vi "Begin.vi"(8 "error in":errorcluster) -> (0 "error out":errorcluster)   [LabVIEW 2018]
doc: "Called before other user functions, this VI is expected to open initial I/O refnums, load in file data, and do all program initialization. Notice that the <B>error out</B> terminal is simply used for data flow. Wiring it to other structures or subVIs ensures that this VI runs first."
uses:
  <vilib>/Rock Robotics/WPI/DriverStation/WPI_DriverStationRobotMode2.ctl
  <vilib>/Rock Robotics/WPI/Joystick/WPI_JoystickDeviceEnum.ctl
  <vilib>/Rock Robotics/WPI/Solenoid/WPI_SolenoidChannel.ctl
  <vilib>/Rock Robotics/WPI/ThirdParty/Phoenix-LabVIEW/Motor Controller/Controls/CTRE_Phoenix_MotorControl_NeutralMode.ctl
  <vilib>/Rock Robotics/WPI/ThirdParty/REV Robotics/SPARK MAX/Typedef/Spark MAX Idle Mode.ctl
  Robot Global Data.vi
  <vilib>/Rock Robotics/Network Tables/NT Write String Array.vi
  <vilib>/Rock Robotics/WPI/Solenoid/WPI_SolenoidOpenDouble.vi
  <vilib>/Rock Robotics/WPI/Solenoid/WPI_SolenoidOpenSingle.vi
  <vilib>/Rock Robotics/WPI/Utilities/WPI_GetSetVariantRefNum.vi
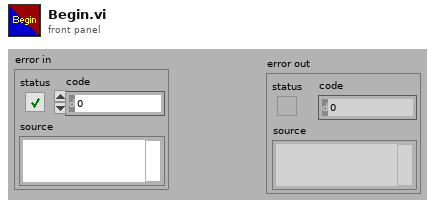
[diagram p1: front panel]
types:
  T1 = typedef "WPI_SolenoidChannel.ctl" = enum8{"Solenoid 0", "Solenoid 1", "Solenoid 2", "Solenoid 3", "Solenoid 4", "Solenoid 5", "Solenoid 6", "Solenoid 7", "Invalid"}
  T2 = typedef "Spark MAX Idle Mode.ctl" = enum16{"Coast", "Brake"}
  T3 = typedef "CTRE_Phoenix_MotorControl_NeutralMode.ctl" = enum8{"EEPROMSetting", "Override to Coast", "Override to Brake"}
  T4 = typedef "WPI_JoystickDeviceEnum.ctl" = enum16{"USB 0", "USB 1", "USB 2", "USB 3", "USB 4", "USB 5"}
  T5 = typedef "WPI_DriverStationRobotMode2.ctl" = enum16{"Autonomous Disabled", "Autonomous Enabled", "Teleop Disabled", "Teleop Enabled", "Disconnected", "Finish", "Test Disabled", "Test Enabled", "Emergency Stopped"}
  T6 = typedef "WPI_JoystickDevRef.ctl" = cluster{"Device":T4}
  T7 = typedef "WPI_MotorControlDeviceRef.ctl" = cluster{"DeviceStatus":errorcluster, "Type":T8, "PWM":cluster{"PWM Channel":T9, "DeadBand":T10}, "CAN":cluster{"Device Number":u8, "SetOutput VI Ref":variant, "GetOutput VI Ref":variant, "Enable VI Ref":variant, "Disable VI Ref":variant, "Data":variant}, "Invert":bool, "DIO PWM":cluster{"PWM \"Enable\" Channel":T9, "DIOChannel":T11, "PWM Rate":dbl}}
  T8 = typedef "WPI_MotorControlType.ctl" = enum16{"PWM", "CAN", "DIO PWM"}
  T9 = typedef "FPGA_DIOPWMChannel.ctl" = enum8{"PWM 0", "PWM 1", "PWM 2", "PWM 3", "PWM 4", "PWM 5", "PWM 6", "PWM 7", "PWM 8", "PWM 9", "PWM MXP 0", "PWM MXP 1", "PWM MXP 2", "PWM MXP 3", "PWM MXP 4", "PWM MXP 5", "PWM MXP 6", "PWM MXP 7", "PWM MXP 8", "PWM MXP 9", "Invalid"}
  T10 = typedef "WPI_PWMDeadband.ctl" = cluster{"Name":string, "maxPositivePwm":i32, "minPositivePwm":i32, "centerPwm":i32, "maxNegativePwm":i32, "minNegativePwm":i32, "angularRange":u16}
  T11 = typedef "FPGA_DIOChannel.ctl" = enum8{"DIO 0", "DIO 1", "DIO 2", "DIO 3", "DIO 4", "DIO 5", "DIO 6", "DIO 7", "DIO 8", "DIO 9", "DIO MXP 0", "DIO MXP 1", "DIO MXP 2", "DIO MXP 3", "DIO MXP 4", "DIO MXP 5", "DIO MXP 6", "DIO MXP 7", "DIO MXP 8", "DIO MXP 9", "DIO MXP 10", "DIO MXP 11", "DIO MXP 12", "DIO MXP 13", "DIO MXP 14", "DIO MXP 15", "SPI Port CS1", "SPI Port CS2", "SPI Port CS3", "SPI Port MISO", "SPI Port MOSI", "Invalid"}
  T12 = typedef "WPI_CompressorDevRef.ctl" = cluster{"DevStatus":errorcluster, "Pneumatics Control Module":u8}
  T13 = typedef "WPI_SolenoidDevRef.ctl" = cluster{"DevStatus":errorcluster, "Pneumatics Control Module":u8, "Forward Solenoid Channel":T1, "Reverse Solenoid Channel":T1}
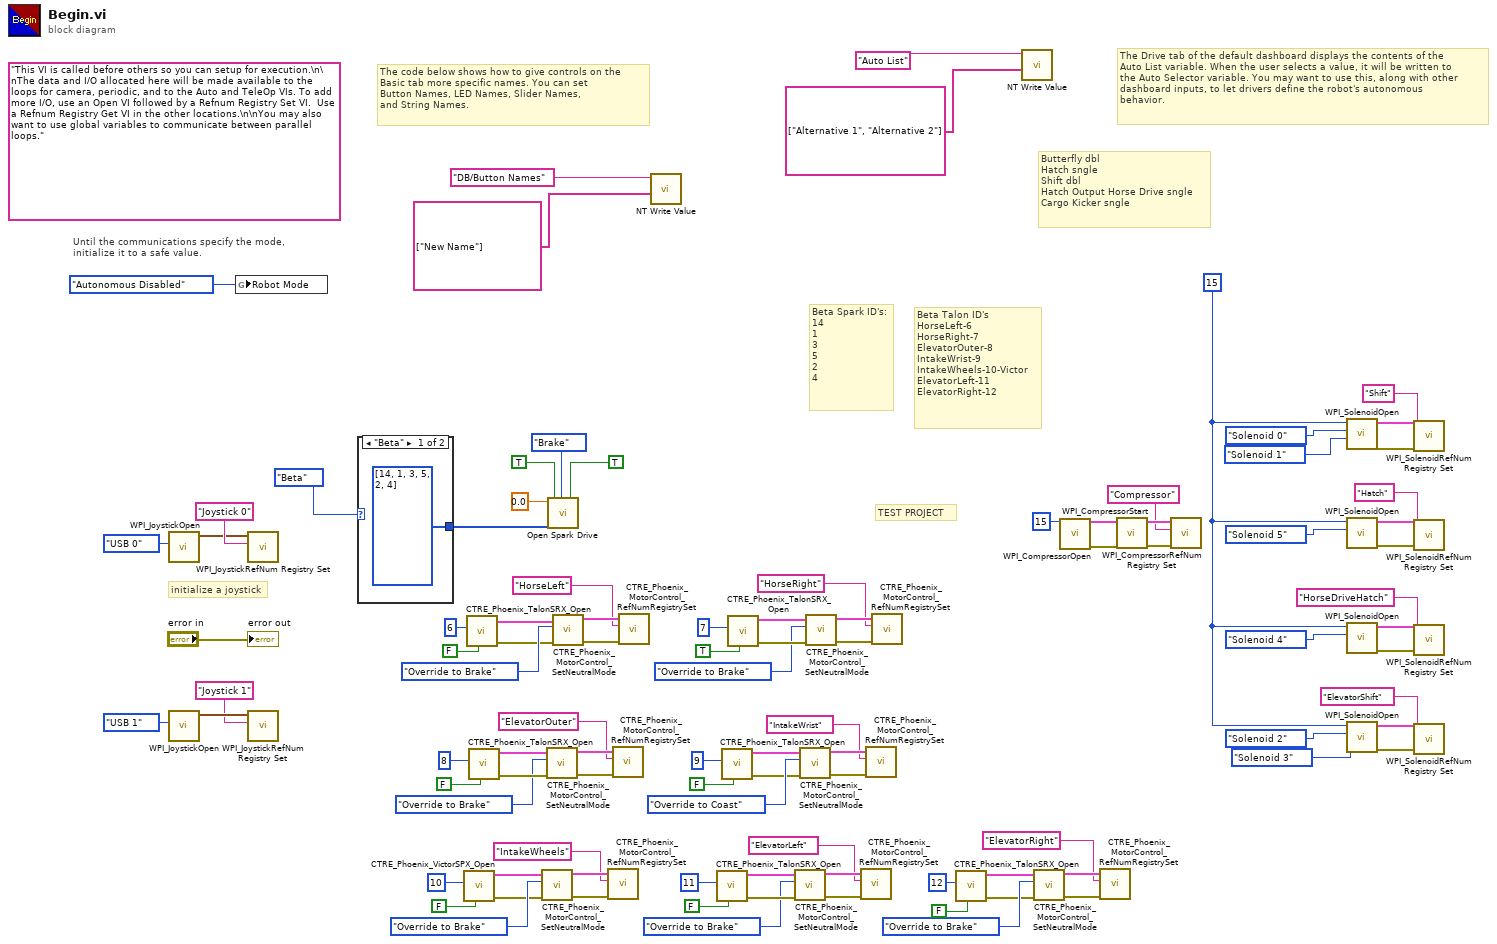
[diagram p0: block diagram]
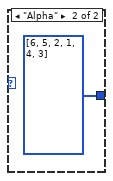
[diagram p2: hidden frame]
diagram:
  w77 = u8 15 ("Pneumatics Control Module (0)")
  (unwired) "This VI is called before others so you can setup for execution.\n\nThe data and I/O allocated here will be made available to the loops for camera, periodic, and to the Auto and TeleOp VIs. To add more I/O, use an Open VI followed by a Refnum Registry Set VI.  Use a Refnum Registry Get VI in the other locations.\n\nYou may also want to use global variables to communicate between parallel loops."
  # "Beta Talon ID's\nHorseLeft-6\nHorseRight-7\nElevatorOuter-8\nIntakeWrist-9\nIntakeWheels-10-Victor\nElevatorLeft-11\nElevatorRight-12"
  # "Beta Spark ID's:\n14\n1\n3\n5\n2\n4"
  # "TEST PROJECT"
  # "Butterfly dbl \nHatch sngle\nShift dbl\nHatch Output Horse Drive sngle\nCargo Kicker sngle"
  # "The Drive tab of the default dashboard displays the contents of the\nAuto List variable. When the user selects a value, it will be written to\nthe Auto Selector variable. You may want to use this, along with other\ndashboard inputs, to let drivers define the robot's autonomous\nbehavior."
  # "The code below shows how to give controls on the\nBasic tab more specific names. You can set\nButton Names, LED Names, Slider Names,\nand String Names."
  # "initialize a joystick"
  # "Until the communications specify the mode,\ninitialize it to a safe value."
  n1 = call <vilib>:"WPI_JoystickOpen.vi"("JoystickDevice"=WPI_JoystickDeviceEnum."USB 0") -> ("JoystickDevRef"=w97:T6)  [unwired: 10 in]
  n2 = call <vilib>:"WPI_JoystickOpen.vi"("JoystickDevice"=WPI_JoystickDeviceEnum."USB 1") -> ("JoystickDevRef"=w75:T6)  [unwired: 10 in]
  n3 = global write "Robot Global Data.vi" "Robot Mode"(WPI_DriverStationRobotMode2."Autonomous Disabled" ("Robot Mode")) -> ()
  n4 = call <vilib>:"WPI_JoystickRefNum Registry Set.vi"("refnum name"="Joystick 0", "JoystickDevRef"=w97) -> ()  [unwired: 8 in, 2 out]
  n5 = call <vilib>:"WPI_JoystickRefNum Registry Set.vi"("refnum name"="Joystick 1", "JoystickDevRef"=w75) -> ()  [unwired: 8 in, 2 out]
  n6 = case shown="\"Beta\"" enum16{"Alpha", "Beta"}."Beta" {
    tunnel: [u8[] [14, 1, 3, 5, 2, 4] ("CAN IDs") u8[] [6, 5, 2, 1, 4, 3] ("CAN IDs")] -> w2
    frame "Beta" {
    }
    frame "Alpha" {
    }
  }
  n7 = call <vilib>:"CTRE_Phoenix_VictorSPX_Open.vi"("Invert"=FALSE, "Device Number"=u8 10) -> ("error out"=w52:errorcluster, "CAN Talon SRX Ref"=w53:T7)  [unwired: 8 in]
  n8 = call <vilib>:"CTRE_Phoenix_TalonSRX_Open.vi"("Invert"=FALSE, "Device Number"=u8 6) -> ("error out"=w18:errorcluster, "CAN Talon SRX Ref"=w19:T7)  [unwired: 8 in]
  n9 = call <vilib>:"CTRE_Phoenix_TalonSRX_Open.vi"("Invert"=FALSE, "Device Number"=u8 8) -> ("error out"=w57:errorcluster, "CAN Talon SRX Ref"=w56:T7)  [unwired: 8 in]
  n10 = call <vilib>:"CTRE_Phoenix_MotorControl_SetNeutralMode.vi"("error in (no error)"=w52, "Motor Control Neutral Mode"=CTRE_Phoenix_MotorControl_NeutralMode."Override to Brake", "PhoenixMotorControlDevRef"=w53) -> ("error out"=w50:errorcluster, "PhoenixMotorControlDevRef"=w51:T7)  [unwired: 7 in]
  n11 = call <vilib>:"CTRE_Phoenix_MotorControl_SetNeutralMode.vi"("error in (no error)"=w57, "Motor Control Neutral Mode"=CTRE_Phoenix_MotorControl_NeutralMode."Override to Brake", "PhoenixMotorControlDevRef"=w56) -> ("error out"=w59:errorcluster, "PhoenixMotorControlDevRef"=w58:T7)  [unwired: 7 in]
  n12 = call "Open Spark Drive.vi"("Set Master/Slave?"=TRUE, "Set Ramp Rate?"=TRUE, "CAN IDs"=w2, "Idle Mode"=Spark_MAX_Idle_Mode."Brake", "Full Acceleration Time"=sgl 0.0 ("Seconds from neutral to full (0)")) -> ()  [unwired: 7 in]
  n13 = call <vilib>:"CTRE_Phoenix_MotorControl_SetNeutralMode.vi"("error in (no error)"=w18, "Motor Control Neutral Mode"=CTRE_Phoenix_MotorControl_NeutralMode."Override to Brake", "PhoenixMotorControlDevRef"=w19) -> ("error out"=w62:errorcluster, "PhoenixMotorControlDevRef"=w63:T7)  [unwired: 7 in]
  n14 = call <vilib>:"CTRE_Phoenix_MotorControl_RefNumRegistrySet.vi"("error in (no error)"=w50, "refnum name"="IntakeWheels" ("string"), "PhoenixMotorControlDevRef"=w51) -> ()  [unwired: 7 in, 2 out]
  n15 = call <vilib>:"CTRE_Phoenix_MotorControl_RefNumRegistrySet.vi"("error in (no error)"=w59, "refnum name"="ElevatorOuter" ("string"), "PhoenixMotorControlDevRef"=w58) -> ()  [unwired: 7 in, 2 out]
  n16 = call <vilib>:"CTRE_Phoenix_MotorControl_RefNumRegistrySet.vi"("error in (no error)"=w62, "refnum name"="HorseLeft" ("string"), "PhoenixMotorControlDevRef"=w63) -> ()  [unwired: 7 in, 2 out]
  n17 = call-poly <vilib>:"NT Write Value.vi"("String Array"=string[] ["New Name"], "Name"="DB/Button Names") -> ()  [unwired: 9 in, 1 out]
  n18 = call <vilib>:"CTRE_Phoenix_TalonSRX_Open.vi"("Invert"=FALSE, "Device Number"=u8 11) -> ("error out"=w43:errorcluster, "CAN Talon SRX Ref"=w42:T7)  [unwired: 8 in]
  n19 = call <vilib>:"CTRE_Phoenix_TalonSRX_Open.vi"("Invert"=FALSE, "Device Number"=u8 9) -> ("error out"=w38:errorcluster, "CAN Talon SRX Ref"=w39:T7)  [unwired: 8 in]
  n20 = call <vilib>:"CTRE_Phoenix_TalonSRX_Open.vi"("Invert"=TRUE, "Device Number"=u8 7) -> ("error out"=w29:errorcluster, "CAN Talon SRX Ref"=w28:T7)  [unwired: 8 in]
  n21 = call <vilib>:"CTRE_Phoenix_MotorControl_SetNeutralMode.vi"("error in (no error)"=w43, "Motor Control Neutral Mode"=CTRE_Phoenix_MotorControl_NeutralMode."Override to Brake", "PhoenixMotorControlDevRef"=w42) -> ("error out"=w45:errorcluster, "PhoenixMotorControlDevRef"=w44:T7)  [unwired: 7 in]
  n22 = call <vilib>:"CTRE_Phoenix_MotorControl_SetNeutralMode.vi"("error in (no error)"=w38, "Motor Control Neutral Mode"=CTRE_Phoenix_MotorControl_NeutralMode."Override to Coast", "PhoenixMotorControlDevRef"=w39) -> ("error out"=w36:errorcluster, "PhoenixMotorControlDevRef"=w37:T7)  [unwired: 7 in]
  n23 = call <vilib>:"CTRE_Phoenix_MotorControl_SetNeutralMode.vi"("error in (no error)"=w29, "Motor Control Neutral Mode"=CTRE_Phoenix_MotorControl_NeutralMode."Override to Brake", "PhoenixMotorControlDevRef"=w28) -> ("error out"=w31:errorcluster, "PhoenixMotorControlDevRef"=w30:T7)  [unwired: 7 in]
  n24 = call <vilib>:"CTRE_Phoenix_MotorControl_RefNumRegistrySet.vi"("error in (no error)"=w45, "refnum name"="ElevatorLeft" ("string"), "PhoenixMotorControlDevRef"=w44) -> ()  [unwired: 7 in, 2 out]
  n25 = call <vilib>:"CTRE_Phoenix_MotorControl_RefNumRegistrySet.vi"("error in (no error)"=w36, "refnum name"="IntakeWrist" ("string"), "PhoenixMotorControlDevRef"=w37) -> ()  [unwired: 7 in, 2 out]
  n26 = call <vilib>:"CTRE_Phoenix_MotorControl_RefNumRegistrySet.vi"("error in (no error)"=w31, "refnum name"="HorseRight" ("string"), "PhoenixMotorControlDevRef"=w30) -> ()  [unwired: 7 in, 2 out]
  n27 = call <vilib>:"CTRE_Phoenix_TalonSRX_Open.vi"("Invert"=FALSE, "Device Number"=u8 12) -> ("error out"=w24:errorcluster, "CAN Talon SRX Ref"=w25:T7)  [unwired: 8 in]
  n28 = call-poly <vilib>:"NT Write Value.vi"("String Array"=string[] ["Alternative 1", "Alternative 2"], "Name"="Auto List") -> ()  [unwired: 9 in, 1 out]
  n29 = call <vilib>:"CTRE_Phoenix_MotorControl_SetNeutralMode.vi"("error in (no error)"=w24, "Motor Control Neutral Mode"=CTRE_Phoenix_MotorControl_NeutralMode."Override to Brake", "PhoenixMotorControlDevRef"=w25) -> ("error out"=w22:errorcluster, "PhoenixMotorControlDevRef"=w23:T7)  [unwired: 7 in]
  n30 = call <vilib>:"WPI_CompressorOpen.vi"("Pneumatics Control Module (0)"=u8 15) -> ("CompressorDevRef"=w69:T12, "error out"=w7:errorcluster)  [unwired: 13 in]
  n31 = call <vilib>:"CTRE_Phoenix_MotorControl_RefNumRegistrySet.vi"("error in (no error)"=w22, "refnum name"="ElevatorRight" ("string"), "PhoenixMotorControlDevRef"=w23) -> ()  [unwired: 7 in, 2 out]
  n32 = call <vilib>:"WPI_CompressorStart.vi"("error in (no error)"=w7, "CompressorDevRef"=w69) -> ("error out"=w67:errorcluster, "CompressorDevRef"=w66:T12)  [unwired: 8 in]
  n33 = call <vilib>:"WPI_CompressorRefNum Registry Set.vi"("error in (no error)"=w67, "refnum name"="Compressor", "CompressorDevRef"=w66) -> ()  [unwired: 7 in, 2 out]
  n34 = call-poly <vilib>:"WPI_SolenoidOpen.vi"("Reverse Solenoid Channel"=WPI_SolenoidChannel."Solenoid 1", "Forward Solenoid Channel"=WPI_SolenoidChannel."Solenoid 0", "Pneumatics Control Module (0)"=w77) -> ("error out"=w73:errorcluster, "SolenoidDevRef"=w87:T13)  [unwired: 7 in]
  n35 = call-poly <vilib>:"WPI_SolenoidOpen.vi"("Solenoid Channel"=WPI_SolenoidChannel."Solenoid 5" ("Forward Solenoid Channel"), "Pneumatics Control Module (0)"=w77) -> ("error out"=w72:errorcluster, "SolenoidDevRef"=w86:T13)  [unwired: 8 in]
  n36 = call-poly <vilib>:"WPI_SolenoidOpen.vi"("Solenoid Channel"=WPI_SolenoidChannel."Solenoid 4" ("Forward Solenoid Channel"), "Pneumatics Control Module (0)"=w77) -> ("error out"=w71:errorcluster, "SolenoidDevRef"=w81:T13)  [unwired: 8 in]
  n37 = call-poly <vilib>:"WPI_SolenoidOpen.vi"("Reverse Solenoid Channel"=WPI_SolenoidChannel."Solenoid 3", "Forward Solenoid Channel"=WPI_SolenoidChannel."Solenoid 2", "Pneumatics Control Module (0)"=w77) -> ("error out"=w70:errorcluster, "SolenoidDevRef"=w80:T13)  [unwired: 7 in]
  n38 = call <vilib>:"WPI_SolenoidRefNum Registry Set.vi"("error in (no error)"=w73, "refnum name"="Shift", "SolenoidDevRef"=w87) -> ()  [unwired: 7 in, 2 out]
  n39 = call <vilib>:"WPI_SolenoidRefNum Registry Set.vi"("error in (no error)"=w72, "refnum name"="Hatch", "SolenoidDevRef"=w86) -> ()  [unwired: 7 in, 2 out]
  n40 = call <vilib>:"WPI_SolenoidRefNum Registry Set.vi"("error in (no error)"=w71, "refnum name"="HorseDriveHatch", "SolenoidDevRef"=w81) -> ()  [unwired: 7 in, 2 out]
  n41 = call <vilib>:"WPI_SolenoidRefNum Registry Set.vi"("error in (no error)"=w70, "refnum name"="ElevatorShift", "SolenoidDevRef"=w80) -> ()  [unwired: 7 in, 2 out]
  "error out" <- "error in"
